vi "doTimeSeries-3D.vi"(0 "period_s":dbl=3600.0, 1 "pixel_dwell_ms":dbl=1.0 caption="Dwell time ms:", 2 "autofocus":bool, 3 "enable":refnum<vi>, 5 "date_stop":timestamp=timestamp(3557127149.3091764 s since 1904-01-01), 7 "pos_start_xyz":T2, 9 "image_size_x_um":dbl=150.0, 11 "frame_size_x_px":i32=100, 12 "pos_start":enum32{"bottom-left", "center"}(ring), 13 "scan_direction":enum32{"0", "1"}(radio)=enum."1" caption="Scan direction:", 14 "IntensityGraph in":refnum<vi>, 15 "z-stack_parameters":T1={"z_start"=0.0, "z_end"=1.0, "z_q_slices"=128, "z-stack_enable"=FALSE} {"z_end" format="%0.2f"; "z_start" format="%0.2f"}) -> ()   [LabVIEW 2014]
panel:
  out "time_remaining":string
  out "image_number":i32
  in  "focus-pixel_dwell_ms":dbl=0.3 caption="focus Dwell time ms:"
  in  "focus-frame_size_x_px":i32=50 caption="frame_size_x_px"
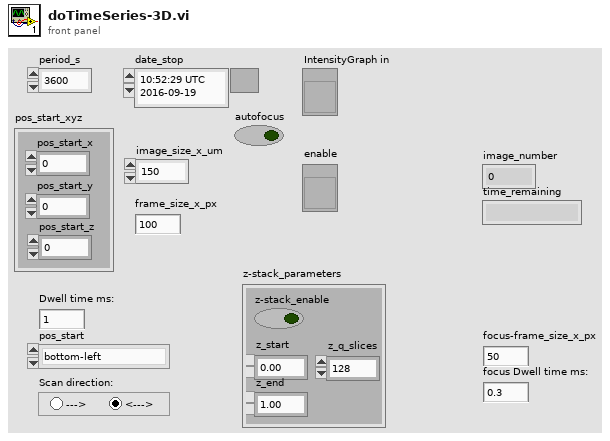
[diagram p1: front panel]
types:
  T1 = cluster{"z_start":dbl, "z_end":dbl, "z_q_slices":i32, "z-stack_enable":bool}
  T2 = cluster{"pos_start_x":dbl, "pos_start_y":dbl, "pos_start_z":dbl}
  T3 = cluster{"image_size_x_um":dbl, "image_size_x_um":dbl}
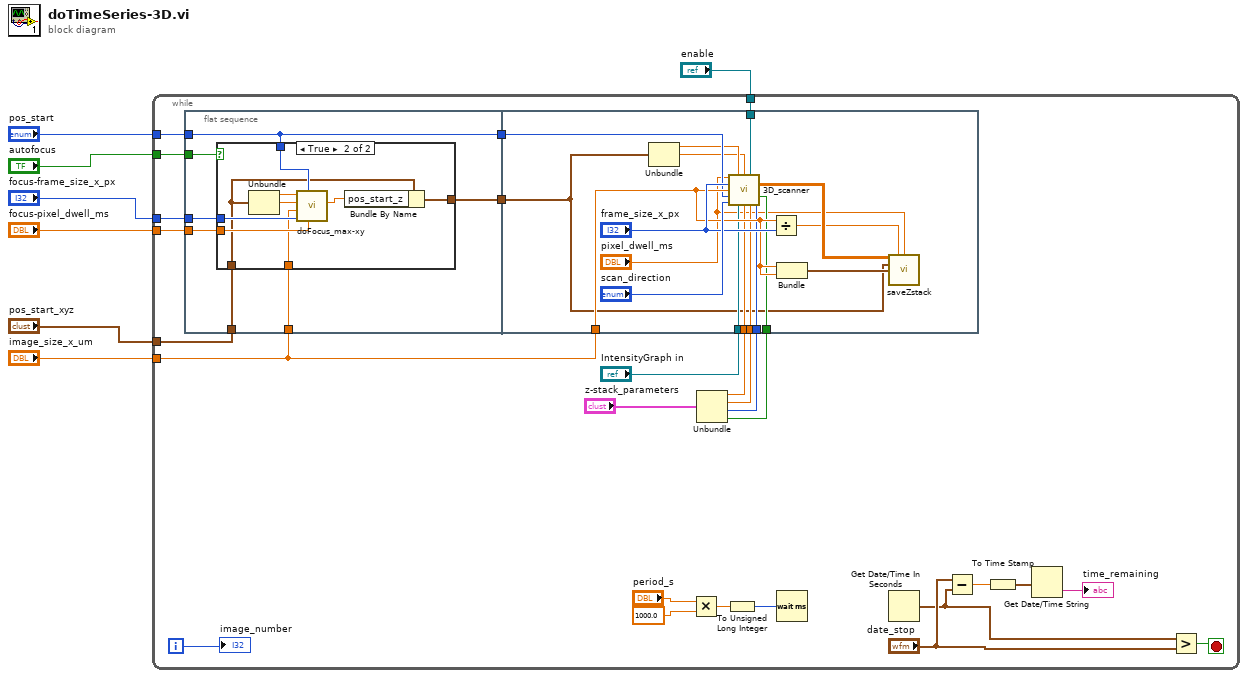
[diagram p0: block diagram]
diagram:
  n1 = while {
    tunnel: "pos_start" -> [w22]
    tunnel: "image_size_x_um" -> [w19]
    tunnel: "autofocus" -> [w23]
    tunnel: "pos_start_xyz" -> [w9]
    tunnel: "focus-pixel_dwell_ms" -> [w21]
    tunnel: "focus-frame_size_x_px" -> [w20]
    tunnel: "enable" -> [w15]
    i -> [w28]
    stop <- w33 stop-if-true
    n2 = flat-sequence {
      tunnel: w23 -> [w40]
      tunnel: w22 -> [w35]
      tunnel: w21 -> [w39]
      tunnel: w20 -> [w38]
      tunnel: w19 -> [w37]
      tunnel: w9 -> [w36]
      tunnel: [w35] -> w17
      tunnel: [w34] -> w8
      tunnel: w19 -> [w65]
      tunnel: w17 -> [w64]
      tunnel: "IntensityGraph in" -> [w61]
      tunnel: w13 -> [w60]
      tunnel: w12 -> [w59]
      tunnel: w11 -> [w58]
      tunnel: w10 -> [w57]
      tunnel: w15 -> [w56]
      tunnel: w8 -> [w51]
      frame #0 {
        n3 = case shown="True" w40 {
          tunnel: w35 -> [_ w50]
          tunnel: w39 -> [_ w49]
          tunnel: w38 -> [_ w48]
          tunnel: w37 -> [_ w47]
          tunnel: w36 -> [w41 w44]
          tunnel: [w41 w42] -> w34
          frame False {
          }
          frame True {
            n4 = Unbundle(w44) -> ("pos_start_x"=w46:dbl, "pos_start_y"=w45:dbl)  [unwired: 1 out]
            n5 = call "doFocus_max-xy.vi"("pixel_dwell_ms"=w49, "pos_start"=w50, "frame_size_x_px"=w48, "image_size_x_um"=w47, "pos-start_y"=w45, "pos-start_x"=w46) -> ("z-focus"=w43:dbl)  [unwired: 4 in, 1 out]
            n6 = Bundle By Name(cluster=w44, "pos_start_z"=w43) -> (w42:T2)
          }
        }
      }
      frame #1 {
        n7 = Unbundle(w51) -> ("pos_start_x"=w63:dbl, "pos_start_y"=w62:dbl)  [unwired: 1 out]
        n8 = call "3D_scanner.vi"("pixel_dwell_ms"="pixel_dwell_ms", "pos-start_x"=w63, "pos-start_y"=w62, "enable"=w56, "frame_size_x_px"="frame_size_x_px", "image_size_x_um"=w65, "pos_start"=w64, "z-stack_enable"=w57, "scan_direction"="scan_direction", "IntensityGraph in"=w61, "z_start"=w60, "z_end"=w59, "z_q_slices"=w58) -> ("image_out"=w55:dbl[][][])  [unwired: 2 in]
        n9 = Divide(x=w65, y="frame_size_x_px") -> (x/y=w53:dbl)
        n10 = Bundle("image_size_x_um"=w65, "image_size_x_um"=w65) -> (w52:T3)  [unwired: 1 in]
        n11 = call "saveZstack.vi"("z-stack_in"=w55, "image-step_size"=w53, "image-dwell_time"="pixel_dwell_ms", "image_start_xyz"=w51, "image_size_xy"=w52) -> ()  [unwired: 11 in]
      }
    }
    n12 = Multiply(x="period_s", y=1000.0) -> (x*y=w30:dbl)
    n13 = Unbundle("z-stack_parameters") -> ("z_start"=w13:dbl, "z_end"=w12:dbl, "z_q_slices"=w11:i32, "z-stack_enable"=w10:bool)
    n14 = To Unsigned Long Integer(number=w30) -> (unsigned 32bit integer=w31:u32)
    n15 = Wait (ms)(milliseconds to wait=w31) -> ()  [unwired: 1 out]
    n16 = Get Date/Time In Seconds() -> (seconds since 1Jan1904=w26:timestamp)
    n17 = Subtract(x="date_stop", y=w26) -> (x-y=w25:dbl)
    n18 = To Time Stamp(1:w25) -> (0:w24:timestamp)
    n19 = Get Date/Time String(seconds (now)=w24) -> (time string=→"time_remaining":string)  [unwired: 2 in, 1 out]
    n20 = Greater?(x=w26, y="date_stop") -> (0:w33:bool)
    "image_number" <- w28
  }
